vi "624WPI_CameraRead MJPEG.vi"(6 "Camera Settings":T2={"fps"=30, "compression"=30, "Image Size"=enum."320x240"}, 8 "Rec Mode":u16(ring) items=["O", "*", "Open Playback Panel"], 9 "Camera IP":string, 10 "Enable":bool, 11 "Refnum in":T1) -> (2 "Active":bool, 3 "Refnum out":T1, 4 "FPS":dbl, 5 "Bandwidth (Mbps)":dbl)   [LabVIEW 2013]
uses:
  <vilib>/Rock Robotics/WPI/Camera/WPI_CameraSettings Read MJPG.ctl
  <vilib>/Rock Robotics/WPI/Camera/WPI_CameraImageSize.ctl
  <vilib>/vision/Image Controls.llb/IMAQ Image.ctl
  <vilib>/Rock Robotics/WPI/Dashboard/WPI_DashboardLogging Global.vi
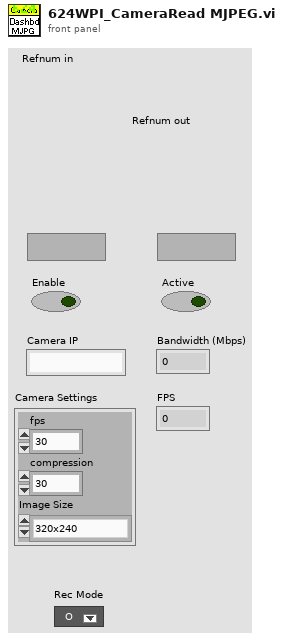
[diagram p1: front panel]
types:
  T1 = typedef "IMAQ Image.ctl" = refnum<image>
  T2 = typedef "WPI_CameraSettings Read MJPG.ctl" = cluster{"fps":i32, "compression":i32, "Image Size":T3}
  T3 = typedef "WPI_CameraImageSize.ctl" = enum16{"640x480", "320x240", "160x120"}
  T4 = typedef "IMAQ AVI2 Refnum.ctl" = refnum<k20>
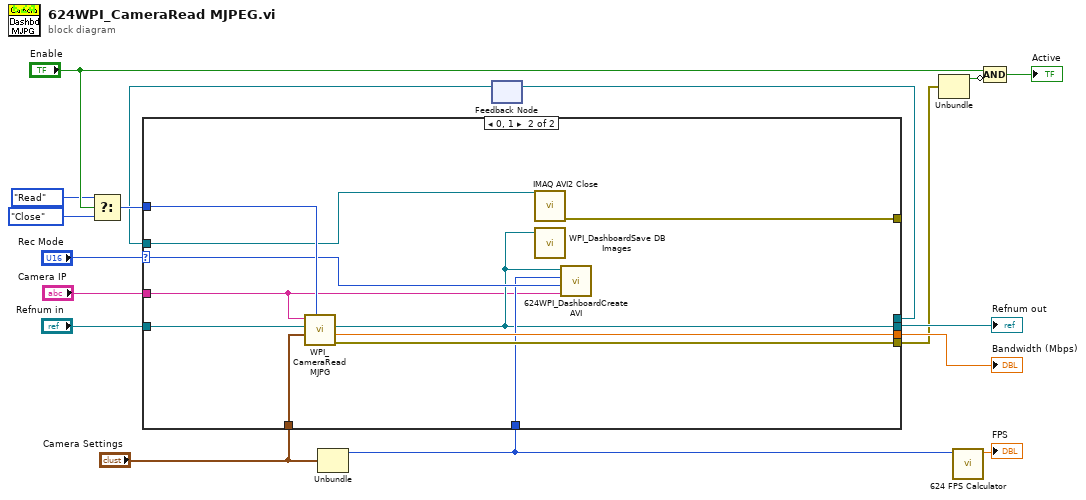
[diagram p0: block diagram]
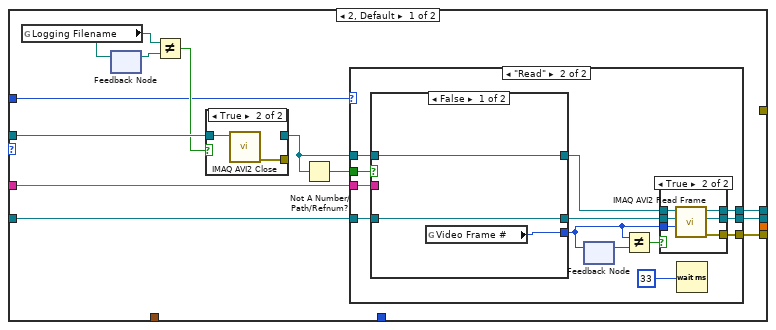
[diagram p2: hidden frame]
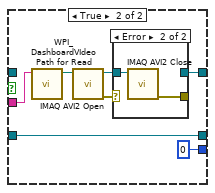
[diagram p5: hidden frame]
diagram:
  n1 = Select(t=enum16{"Read", "Reopen", "Close"}."Read" ("Operation"), s="Enable", f=enum16{"Read", "Reopen", "Close"}."Close" ("Operation")) -> (s? t:f=w13:enum16{"Read", "Reopen", "Close"})
  n2 = Unbundle("Camera Settings") -> ("fps"=w2:i32)  [unwired: 2 out]
  n3 = feedback #1() -> (w5:T4)  [unwired: 1 in]
  n4 = case shown="0, 1" "Rec Mode" {
    selector: "Rec Mode" -> [_ w72]
    tunnel: "Camera Settings" -> [_ w79]
    tunnel: w13 -> [w18 w78]
    tunnel: [_ w77] -> w10
    tunnel: [w29 w70] -> w6
    tunnel: "Refnum in" -> [w27 w76]
    tunnel: "Camera IP" -> [w24 w69]
    tunnel: w2 -> [_ w71]
    tunnel: w5 -> [w22 w74]
    tunnel: [w26 _] -> w4
    tunnel: [w25 w75] -> w3
    tunnel: [_ w73] -> _
    frame 2, Default {
      n5 = global read "WPI_DashboardLogging Global.vi" "Logging Filename"() -> (w21:path)
      n6 = feedback #2() -> (w20:path)  [unwired: 1 in]
      n7 = feedback-in #2(w21) -> ()
      n8 = Not Equal?(x=w21, y=w20) -> (x != y?=w19:bool)
      n9 = case shown="True" w19 {
        tunnel: [w66 _] -> w23
        tunnel: w22 -> [w66 w68]
        tunnel: [_ w67] -> _
        frame False {
        }
        frame True {
          n10 = call "IMAQ AVI2 Close"("AVI Refnum"=w68) -> ("error out"=w67:errorcluster)  [unwired: 10 in]
        }
      }
      n11 = Not A Number/Path/Refnum?(number/path/refnum=w23) -> (NaN/Path/Refnum?=w28:bool)
      n12 = case shown="\"Read\"" w18 {
        tunnel: [w30 w44] -> w29
        tunnel: w28 -> [_ w43]
        tunnel: w27 -> [w30 w40]
        tunnel: [w31 w39] -> w26
        tunnel: [_ w38] -> w25
        tunnel: w24 -> [_ w37]
        tunnel: w23 -> [w31 w36]
        frame "Close", Default {
        }
        frame "Read" {
          n13 = case shown="False" w43 {
            tunnel: [w55 w60] -> w42
            tunnel: w36 -> [w55 _]
            tunnel: [w54 w62] -> w41
            tunnel: w40 -> [w54 w62]
            tunnel: [w53 0 ("Video Frame #")] -> w33
            tunnel: w37 -> [_ w57]
            frame False {
              n14 = global read "WPI_DashboardLogging Global.vi" "Video Frame #"() -> (w53:i32)
            }
            frame True {
              n15 = call <vilib>:"WPI_DashboardVIdeo Path for Read.vi"("Camera IP"=w57) -> ("Video Path"=w56:path)  [unwired: 10 in]
              n16 = call "IMAQ AVI2 Open"("AVI File Path"=w56) -> ("error out"=w61:errorcluster, "AVI Refnum"=w59:T4)  [unwired: 9 in]
              n17 = case shown="Error" w61 {
                tunnel: [w63 _] -> w60
                tunnel: w59 -> [w63 w65]
                tunnel: [_ w64] -> _
                frame No Error {
                }
                frame Error {
                  n18 = call "IMAQ AVI2 Close"("AVI Refnum"=w65) -> ("error out"=w64:errorcluster)  [unwired: 10 in]
                }
              }
            }
          }
          n19 = feedback #3() -> (w34:i32)  [unwired: 1 in]
          n20 = feedback-in #3(w33) -> ()
          n21 = Not Equal?(x=w33, y=w34) -> (x != y?=w35:bool)
          n22 = case shown="True" w35 {
            tunnel: [w45 w52] -> w44
            tunnel: w42 -> [w46 w51]
            tunnel: w41 -> [w45 w50]
            tunnel: [w46 w49] -> w39
            tunnel: [_ w48] -> w38
            tunnel: w33 -> [_ w47]
            frame False {
            }
            frame True {
              n23 = call "IMAQ AVI2 Read Frame"("Frame Number"=w47, "Image"=w50, "AVI Refnum"=w51) -> ("error out"=w48:errorcluster, "Image Out"=w52:T1, "AVI Refnum (duplicate)"=w49:T4)  [unwired: 6 in]
            }
          }
          n24 = Wait (ms)(milliseconds to wait=33) -> ()  [unwired: 1 out]
        }
      }
    }
    frame 0, 1 {
      n25 = call <vilib>:"WPI_CameraRead MJPG.vi"("Operation"=w78, "Camera Settings"=w79, "Image"=w76, "address"=w69) -> ("error out"=w75:errorcluster, "Bandwidth (Mbps)"=w77:dbl, "Image Out"=w70:T1)  [unwired: 5 in]
      n26 = call "IMAQ AVI2 Close"("AVI Refnum"=w74) -> ("error out"=w73:errorcluster)  [unwired: 10 in]
      n27 = call <vilib>:"WPI_DashboardSave DB Images.vi"("Image"=w70) -> ()  [unwired: 3 in]
      n28 = call "624WPI_DashboardCreate AVI.vi"("Camera IP"=w69, "Recording"=w72, "frames per seconds"=w71, "Image"=w70) -> ()  [unwired: 8 in]
    }
  }
  "Bandwidth (Mbps)" <- w10
  "Refnum out" <- w6
  n29 = feedback-in #1(w4) -> ()
  n30 = Unbundle(w3) -> ("status"=w15:bool)  [unwired: 2 out]
  n31 = call "624 FPS Calculator.vi"("Average Count"=w2) -> ("fps"=→"FPS":dbl)  [unwired: 10 in]
  n32 = Compound Arithmetic op=AND("Enable", invert w15) -> (→"Active":bool)
